vi "isolate_common_trigger.vi"(8 "error in (no error)":errorcluster, 10 "trigger variant in":variant, 11 "GenericToplevelComponent in":refnum<class "GenericToplevelComponent.lvclass">) -> (0 "error out":errorcluster, 1 "common trigger":T2, 2 "trigger variant out":variant, 3 "GenericToplevelComponent out":refnum<class "GenericToplevelComponent.lvclass">, 4 "is common trigger?":bool, 6 "trigger type":T1)   [LabVIEW 2010, in "GenericToplevelComponent.lvclass"]
uses:
  GenericToplevelComponent.lvclass
  common_trigger_enum.ctl
  trigger_type_enum.ctl
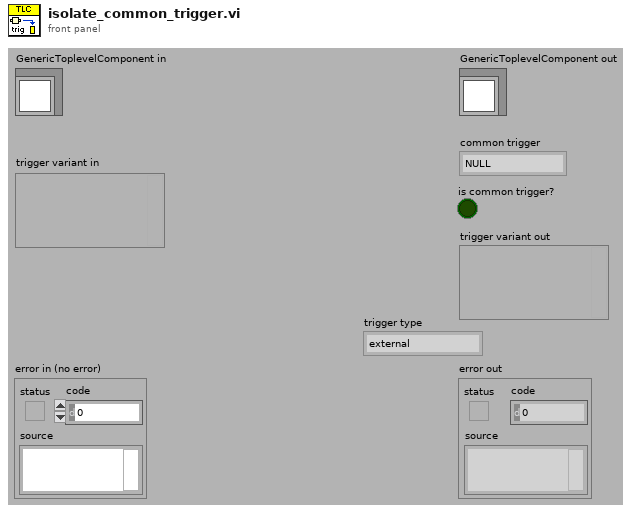
[diagram p1: front panel]
types:
  T1 = typedef "trigger_type_enum.ctl" = enum8{"external", "internal", "common"}
  T2 = typedef "GenericToplevelComponent.lvclass/common_trigger_enum.ctl" = enum16{"NULL", "initialise", "terminate", "fetch command", "fetch data", "register as observer"}
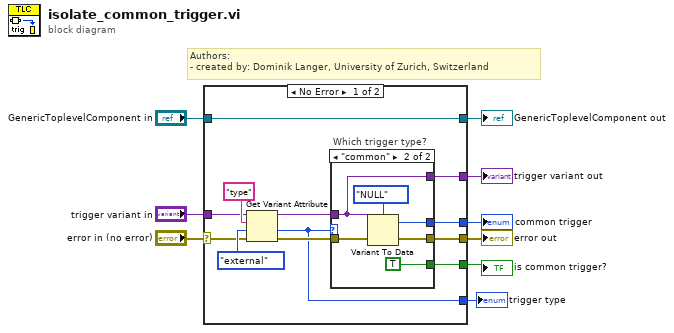
[diagram p0: block diagram]
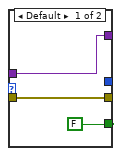
[diagram p2: hidden frame]
diagram:
  # "Authors: \n- created by: Dominik Langer, University of Zurich, Switzerland"
  n1 = case shown="No Error" "error in (no error)" {
    selector: "error in (no error)" -> [w18 w33]
    tunnel: [w15 w33] -> w8
    tunnel: [w21 w32] -> w6
    tunnel: "GenericToplevelComponent in" -> [w21 w32]
    tunnel: "trigger variant in" -> [w17 w31]
    tunnel: [w13 w31] -> w4
    tunnel: [w12 _] -> w3
    tunnel: [w11 _] -> w2
    tunnel: [w10 _] -> w1
    frame No Error {
      n2 = Get Variant Attribute(Variant=w17, name="type", default value (empty Variant)=trigger_type_enum."external" ("trigger type"), error in=w18) -> (duplicate Variant=w14:variant, value=w10:T1, error out=w16:errorcluster)  [unwired: 1 out]
      n3 = case "Which trigger type?" shown="\"common\"" w10 {
        tunnel: w16 -> [w24 w30]
        tunnel: [w24 w29] -> w15
        tunnel: w14 -> [w23 w27]
        tunnel: [w23 w27] -> w13
        tunnel: [_ w26] -> w12
        tunnel: [FALSE TRUE] -> w11
        frame Default {
        }
        frame "common" {
          n4 = Variant To Data(error in=w30, Variant=w27, type=common_trigger_enum."NULL" ("trigger")) -> (error out=w29:errorcluster, data=w26:T2)
        }
      }
    }
    frame Error {
    }
  }
  "error out" <- w8
  "GenericToplevelComponent out" <- w6
  "trigger variant out" <- w4
  "common trigger" <- w3
  "is common trigger?" <- w2
  "trigger type" <- w1
